vi "NavbalLabVIEW(15-5-21).vi"() -> ()   [LabVIEW 2010] (continued)
              n791 = Increment(x=w3724) -> (x+1=w3725:i32)
              n792 = local read "#Corner Accels"() -> (w3709:i32)
              n793 = Add(x=w3718, y=w3719) -> (x+y=w3720:i32)
              n794 = Add(x=12, y=w3720) -> (x+y=w3722:i32)
              n795 = Decrement(x=w3722) -> (x-1=w3717:i32)
              n796 = Bundle(w3717, w3725) -> (w3730:cluster{i32, i32})  [unwired: 1 in]
              n797 = call-poly <vilib>:"Excel Get Data.vi"("report in"=w3737, "data type"=string[][] [], "start (-1, -1)"=w3731, "end (-1, -1)"=w3730, "error in (no error)"=w3738) -> ("data"=w3729:string[][], "error out"=w3723:errorcluster)  [unwired: 9 out]
              n798 = call <vilib>:"General Error Handler.vi"("error in (no error)"=w3723) -> ()  [unwired: 2 in, 13 out]
              n799 = Fract/Exp String To Number(string=w3729) -> (number=w3710:dbl[][])  [unwired: 3 in, 1 out]
              n800 = case shown="\"Port Side\", Default" w3711 {
                tunnel: w3710 -> [w3752 w3766]
                tunnel: [w3744 w3757] -> w3712
                tunnel: w3709 -> [w3741 w3756]
                frame "Port Side", Default {
                  n801 = Initialize Array(0.0 ("element"), w3741, 2 ("dimension size")) -> (w3749:dbl[][])
                  n802 = Insert Into Array(array=w3752, index (row)=0, new element=w3749) -> (w3748:dbl[][])  [unwired: 1 in]
                  n803 = Multiply(x=2, y=w3741) -> (x*y=w3740:i32)
                  n804 = local read "#Stbd Accels"() -> (w3739:i32)
                  n805 = Initialize Array(0.0 ("element"), w3739, 2 ("dimension size")) -> (w3745:dbl[][])
                  n806 = Insert Into Array(array=w3748, index (row)=w3740, new element=w3745) -> (w3744:dbl[][])  [unwired: 1 in]
                }
                frame "Stbd Side" {
                  n807 = local read "#Stbd Accels"() -> (w3753:i32)
                  n808 = Initialize Array(0.0 ("element"), w3756, 2 ("dimension size")) -> (w3763:dbl[][])
                  n809 = Insert Into Array(array=w3766, index (row)=w3756, new element=w3763) -> (w3762:dbl[][])  [unwired: 1 in]
                  n810 = Multiply(x=2, y=w3756) -> (x*y=w3754:i32)
                  n811 = Add(x=w3754, y=w3753) -> (x+y=w3761:i32)
                  n812 = Initialize Array(0.0 ("element"), w3753, 2 ("dimension size")) -> (w3758:dbl[][])
                  n813 = Insert Into Array(array=w3762, index (row)=w3761, new element=w3758) -> (w3757:dbl[][])  [unwired: 1 in]
                }
              }
              "Ref Pt Plot" <- w3712
            }
          }
          n814 = case shown="True" "Refresh Plot Listbox" {
            tunnel: w3337 -> [_ w3779]
            frame False {
            }
            frame True {
              n815 = local read "Port/Starboard"() -> (w3782:enum32{"Port Side", "Stbd Side"})
              n816 = case shown="\"Port Side\", Default" w3782 {
                tunnel: ["Data-Port" "Data-Stbd"] -> w3781
                frame "Port Side", Default {
                }
                frame "Stbd Side" {
                }
              }
              n817 = call <vilib>:"New Report.vi"("report type"=T11."Excel", "template (empty)"=w3779) -> ("report out"=w3785:refnum<class "NI_report.lvclass">, "error out"=w3784:errorcluster)  [unwired: 12 in]
              n818 = call <vilib>:"Excel Get Worksheet.vi"("report in"=w3785, "error in (no error)"=w3784, "name (\"\")"=w3781) -> ("report out"=w3798:refnum<class "NI_report.lvclass">, "error out"=w3797:errorcluster)  [unwired: 1 in, 10 out]
              n819 = Increment(x="# Runs") -> (x+1=w3786:dbl)
              n820 = Multiply(x=w3786, y=2) -> (x*y=w3788:dbl)
              n821 = Bundle("row"=2, w3788) -> (w3787:cluster{"row":i32, dbl})  [unwired: 1 in]
              n822 = call-poly <vilib>:"Excel Get Data.vi"("report in"=w3798, "data type"=string[][] [], "start (-1, -1)"=cluster{"row":i32, "column":i32} {"row"=0, "column"=1}, "end (-1, -1)"=w3787, "error in (no error)"=w3797) -> ("data"=w3792:string[][])  [unwired: 10 out]
              n823 = Transpose 2D Array(2D array=w3792) -> (transposed array=w3795:string[][])
              n824 = local read "Predicted Phase"() -> (w3775:dbl[])
              n825 = Index Array(array=w3795, index (col)=0 ("disabled index (col)")) -> (element=w3794:string[])  [unwired: 1 in]
              n826 = Decimate 1D Array(w3794) -> (w3791:string[])  [unwired: 1 out]
              n827 = Array Size(array=w3791) -> (size(s)=w3793:i32)
              n828 = Reshape Array(w3791, w3793, 1 ("dimension size")) -> (w3783:string[][])
              n829 = local read "Predicted Mag"() -> (w3776:dbl[])
              n830 = local read "Select Side to Analyze"() -> (w3771:enum32{"Starboard", "Port"})
              n831 = property on="Marker Listbox" class="MCListbox (strict)"("ItemNames"=w3783) -> ()  [unwired: 2 in, 2 out]
              n832 = local read "#Corner Accels"() -> (w3773:i32)
              n833 = Build Array(w3776, w3775) -> (w3777:dbl[][])
              n834 = Transpose 2D Array(2D array=w3777) -> (transposed array=w3774:dbl[][])
              n835 = case shown="\"Port\"" w3771 {
                tunnel: w3774 -> [w3815 w3829]
                tunnel: [w3806 w3821] -> w3772
                tunnel: w3773 -> [w3805 w3818]
                frame "Starboard", Default {
                  n836 = local read "#Stbd Accels"() -> (w3802:i32)
                  n837 = Initialize Array(0.0 ("element"), w3805, 2 ("dimension size")) -> (w3812:dbl[][])
                  n838 = Insert Into Array(array=w3815, index (row)=w3805, new element=w3812) -> (w3811:dbl[][])  [unwired: 1 in]
                  n839 = Multiply(x=2, y=w3805) -> (x*y=w3803:i32)
                  n840 = Add(x=w3803, y=w3802) -> (x+y=w3810:i32)
                  n841 = Initialize Array(0.0 ("element"), w3802, 2 ("dimension size")) -> (w3807:dbl[][])
                  n842 = Insert Into Array(array=w3811, index (row)=w3810, new element=w3807) -> (w3806:dbl[][])  [unwired: 1 in]
                }
                frame "Port" {
                  n843 = Initialize Array(0.0 ("element"), w3818, 2 ("dimension size")) -> (w3826:dbl[][])
                  n844 = Insert Into Array(array=w3829, index (row)=0, new element=w3826) -> (w3825:dbl[][])  [unwired: 1 in]
                  n845 = Multiply(x=2, y=w3818) -> (x*y=w3817:i32)
                  n846 = local read "#Stbd Accels"() -> (w3816:i32)
                  n847 = Initialize Array(0.0 ("element"), w3816, 2 ("dimension size")) -> (w3822:dbl[][])
                  n848 = Insert Into Array(array=w3825, index (row)=w3817, new element=w3822) -> (w3821:dbl[][])  [unwired: 1 in]
                }
              }
              "Pred plot" <- w3772
            }
          }
          n849 = Divide(x=159.0, y=w3556) -> (x/y=w3700:dbl)
          n850 = Divide(x=159.0, y=w3557) -> (x/y=w3685:dbl)
          n851 = Logarithm Base 10(1:w3700) -> (0:w3699:dbl)
          n852 = Divide(x=159.0, y=w3643) -> (x/y=w3658:dbl)
          n853 = Logarithm Base 10(1:w3685) -> (0:w3684:dbl)
          n854 = Divide(x=159.0, y=w3483) -> (x/y=w3509:dbl)
          n855 = Multiply(x=20.0, y=w3699) -> (x*y=w3698:dbl)
          n856 = Logarithm Base 10(1:w3658) -> (0:w3657:dbl)
          n857 = Multiply(x=20.0, y=w3684) -> (x*y=w3683:dbl)
          n858 = Logarithm Base 10(1:w3509) -> (0:w3508:dbl)
          n859 = Subtract(x=w3696, y=w3698) -> (x-y=w3692:dbl[][])
          "Magnitude AdB Stbd" <- w3692
          n860 = Multiply(x=20.0, y=w3657) -> (x*y=w3656:dbl)
          n861 = Subtract(x=w3681, y=w3683) -> (x-y=w3674:dbl[][])
          "Magnitude AdB Port" <- w3674
          n862 = Multiply(x=20.0, y=w3508) -> (x*y=w3507:dbl)
          n863 = Subtract(x=w3644, y=w3656) -> (x-y=w3642:dbl[][])
          "Magnitude AdB Corner" <- w3642
          n864 = Subtract(x=w3495, y=w3507) -> (x-y=w3494:dbl[][])
          "Magnitude AdB Corners-Port" <- w3494
          n865 = local read "Averaging"() -> (w3365:bool)
          n866 = for "Mils(8x)" {
            N: w3521 -> [_]
            tunnel: w3696 -> [w5009]
            tunnel: w3556 -> [w5005]
            tunnel: [w5004] -> w3639 mode=indexing
            tunnel: [w5003] -> w3697 mode=indexing
            i -> [w5006]
            n867 = Index Array(array=w5009, index (row)=w5006) -> (element=w5007:dbl[])  [unwired: 1 in]
            n868 = for {
              N: 8 -> [_]
              tunnel: w5007 -> [w5018]
              tunnel: w5005 -> [w5026]
              tunnel: [w5012] -> w5004 mode=indexing
              tunnel: [w5010] -> w5003 mode=indexing
              i -> [w5025]
              n869 = Add(x=w5025, y=1) -> (x+y=w5027:i32)
              n870 = Index Array(array=w5018, index=w5025) -> (element=w5019:dbl)
              n871 = Multiply(x=w5026, y=w5027) -> (x*y=w5010:dbl)
              n872 = Divide(x=159, y=w5010) -> (x/y=w5023:dbl)
              n873 = Logarithm Base 10(1:w5023) -> (0:w5022:dbl)
              n874 = Multiply(x=20.0, y=w5022) -> (x*y=w5020:dbl)
              n875 = Subtract(x=w5019, y=w5020) -> (x-y=w5013:dbl)
              n876 = Divide(x=w5013, y=20.0) -> (x/y=w5015:dbl)
              n877 = Power Of 10(x=w5015) -> (10^x=w5017:dbl)
              n878 = Multiply(x=w5017, y=0.0887) -> (x*y=w5011:dbl)
              n879 = Divide(x=w5011, y=w5010) -> (x/y=w5012:dbl)
            }
          }
          "Mils/sec Stbd" <- w3639
          "Freq Stbd" <- w3697
          n880 = for "Mils(8x)" {
            N: w3519 -> [_]
            tunnel: w3681 -> [w4901]
            tunnel: w3557 -> [w4897]
            tunnel: [w4896] -> w3619 mode=indexing
            tunnel: [w4895] -> w3682 mode=indexing
            i -> [w4898]
            n881 = Index Array(array=w4901, index (row)=w4898) -> (element=w4899:dbl[])  [unwired: 1 in]
            n882 = for {
              N: 8 -> [_]
              tunnel: w4899 -> [w4910]
              tunnel: w4897 -> [w4918]
              tunnel: [w4904] -> w4896 mode=indexing
              tunnel: [w4902] -> w4895 mode=indexing
              i -> [w4917]
              n883 = Add(x=w4917, y=1) -> (x+y=w4919:i32)
              n884 = Index Array(array=w4910, index=w4917) -> (element=w4911:dbl)
              n885 = Multiply(x=w4918, y=w4919) -> (x*y=w4902:dbl)
              n886 = Divide(x=159, y=w4902) -> (x/y=w4915:dbl)
              n887 = Logarithm Base 10(1:w4915) -> (0:w4914:dbl)
              n888 = Multiply(x=20.0, y=w4914) -> (x*y=w4912:dbl)
              n889 = Subtract(x=w4911, y=w4912) -> (x-y=w4905:dbl)
              n890 = Divide(x=w4905, y=20.0) -> (x/y=w4907:dbl)
              n891 = Power Of 10(x=w4907) -> (10^x=w4909:dbl)
              n892 = Multiply(x=w4909, y=0.0887) -> (x*y=w4903:dbl)
              n893 = Divide(x=w4903, y=w4902) -> (x/y=w4904:dbl)
            }
          }
          "Mils/sec Port" <- w3619
          "Freq Port" <- w3682
          n894 = Index Array(array=w3692, index (col)=0 ("disabled index (col)")) -> (element=w3693:dbl[])  [unwired: 1 in]
          n895 = local read "Averaging"() -> (w3358:bool)
          n896 = for "Mils(8x)" {
            N: w3571 -> [_]
            tunnel: w3644 -> [w4713]
            tunnel: w3643 -> [w4709]
            tunnel: [w4708] -> w3617 mode=indexing
            tunnel: [w4707] -> w3655 mode=indexing
            i -> [w4710]
            n897 = Index Array(array=w4713, index (row)=w4710) -> (element=w4711:dbl[])  [unwired: 1 in]
            n898 = for {
              N: 8 -> [_]
              tunnel: w4711 -> [w4722]
              tunnel: w4709 -> [w4730]
              tunnel: [w4716] -> w4708 mode=indexing
              tunnel: [w4714] -> w4707 mode=indexing
              i -> [w4729]
              n899 = Add(x=w4729, y=1) -> (x+y=w4731:i32)
              n900 = Index Array(array=w4722, index=w4729) -> (element=w4723:dbl)
              n901 = Multiply(x=w4730, y=w4731) -> (x*y=w4714:dbl)
              n902 = Divide(x=159, y=w4714) -> (x/y=w4727:dbl)
              n903 = Logarithm Base 10(1:w4727) -> (0:w4726:dbl)
              n904 = Multiply(x=20.0, y=w4726) -> (x*y=w4724:dbl)
              n905 = Subtract(x=w4723, y=w4724) -> (x-y=w4717:dbl)
              n906 = Divide(x=w4717, y=20.0) -> (x/y=w4719:dbl)
              n907 = Power Of 10(x=w4719) -> (10^x=w4721:dbl)
              n908 = Multiply(x=w4721, y=0.0887) -> (x*y=w4715:dbl)
              n909 = Divide(x=w4715, y=w4714) -> (x/y=w4716:dbl)
            }
          }
          "Mils/sec Corner" <- w3617
          "Freq Corner" <- w3655
          n910 = Index Array(array=w3674, index (col)=0 ("disabled index (col)")) -> (element=w3678:dbl[])  [unwired: 1 in]
          n911 = for "Mils(8x)" {
            N: w3481 -> [_]
            tunnel: w3495 -> [w4264]
            tunnel: w3483 -> [w4260]
            tunnel: [w4259] -> w3485 mode=indexing
            tunnel: [w4258] -> w3506 mode=indexing
            i -> [w4261]
            n912 = Index Array(array=w4264, index (row)=w4261) -> (element=w4262:dbl[])  [unwired: 1 in]
            n913 = for {
              N: 8 -> [_]
              tunnel: w4262 -> [w4273]
              tunnel: w4260 -> [w4281]
              tunnel: [w4267] -> w4259 mode=indexing
              tunnel: [w4265] -> w4258 mode=indexing
              i -> [w4280]
              n914 = Add(x=w4280, y=1) -> (x+y=w4282:i32)
              n915 = Index Array(array=w4273, index=w4280) -> (element=w4274:dbl)
              n916 = Multiply(x=w4281, y=w4282) -> (x*y=w4265:dbl)
              n917 = Divide(x=159, y=w4265) -> (x/y=w4278:dbl)
              n918 = Logarithm Base 10(1:w4278) -> (0:w4277:dbl)
              n919 = Multiply(x=20.0, y=w4277) -> (x*y=w4275:dbl)
              n920 = Subtract(x=w4274, y=w4275) -> (x-y=w4268:dbl)
              n921 = Divide(x=w4268, y=20.0) -> (x/y=w4270:dbl)
              n922 = Power Of 10(x=w4270) -> (10^x=w4272:dbl)
              n923 = Multiply(x=w4272, y=0.0887) -> (x*y=w4266:dbl)
              n924 = Divide(x=w4266, y=w4265) -> (x/y=w4267:dbl)
            }
          }
          "Mils/sec Corners-Port" <- w3485
          "Freq Corner Port" <- w3506
          n925 = local read "Averaging"() -> (w3356:bool)
          n926 = local read "Averaging"() -> (w3357:bool)
          n927 = Index Array(array=w3642, index (col)=0 ("disabled index (col)")) -> (element=w3652:dbl[])  [unwired: 1 in]
          n928 = Array Size(array=w3693) -> (size(s)=w3695:i32)
          n929 = Index Array(array=w3494, index (col)=0 ("disabled index (col)")) -> (element=w3503:dbl[])  [unwired: 1 in]
          n930 = Index Array(array=w3639, index (col)=0 ("index (row)")) -> (element=w3363:dbl[])  [unwired: 1 in]
          n931 = Index Array(array=w3558, index (col)=0 ("index")) -> (element=w3364:dbl[])  [unwired: 1 in]
          n932 = Index Array(array=w3692, index (col)=0 ("index (row)")) -> (element=w3361:dbl[])  [unwired: 1 in]
          n933 = Array Size(array=w3678) -> (size(s)=w3680:i32)
          n934 = Index Array(array=w3619, index (col)=0 ("index (row)")) -> (element=w3675:dbl[])  [unwired: 1 in]
          n935 = case shown="True" w3365 {
            tunnel: [w3879 w3880] -> w3362
            tunnel: w3364 -> [w3879 w3881]
            frame False {
            }
            frame True {
              n936 = call "Time Averaging3"("input signals"=w3881) -> ("time avg. signal"=w3880:dbl[])  [unwired: 15 in, 3 out]
            }
          }
          n937 = Index Array(array=w3415, index (col)=0 ("index")) -> (element=w3414:dbl[])  [unwired: 1 in]
          n938 = Index Array(array=w3674, index (col)=0 ("index (row)")) -> (element=w3673:dbl[])  [unwired: 1 in]
          n939 = Array Size(array=w3652) -> (size(s)=w3654:i32)
          n940 = for "Mils(1x)" {
            N: w3695 -> [_]
            tunnel: w3556 -> [w4998]
            tunnel: [w4993] -> w3360 mode=indexing
            tunnel: w3693 -> [w4992]
            i -> [w5002]
            n941 = Square(x=w4998) -> (x^2=w4996:dbl)
            n942 = Index Array(array=w4992, index #1=w5002) -> (element #1=w5001:dbl)  [unwired: 1 in, 1 out]
            n943 = Divide(x=0.028175, y=w4996) -> (x/y=w4994:dbl)
            n944 = Divide(x=w5001, y=20.0) -> (x/y=w4999:dbl)
            n945 = Power Of 10(x=w4999) -> (10^x=w4995:dbl)
            n946 = Multiply(x=w4995, y=w4994) -> (x*y=w4993:dbl)
          }
          "Mils(1x) Stbd" <- w3360
          n947 = case shown="True" w3358 {
            tunnel: w3414 -> [w3876 w3878]
            tunnel: [w3876 w3877] -> w3408
            frame False {
            }
            frame True {
              n948 = call "Time Averaging2"("input signals"=w3878) -> ("time avg. signal"=w3877:dbl[])  [unwired: 15 in, 3 out]
            }
          }
          n949 = Index Array(array=w3617, index (col)=0 ("index (row)")) -> (element=w3649:dbl[])  [unwired: 1 in]
          n950 = Index Array(array=w3618, index (col)=0 ("index")) -> (element=w3413:dbl[])  [unwired: 1 in]
          n951 = Index Array(array=w3642, index (col)=0 ("index (row)")) -> (element=w3648:dbl[])  [unwired: 1 in]
          n952 = Array Size(array=w3503) -> (size(s)=w3505:i32)
          n953 = for "Mils(1x)" {
            N: w3680 -> [_]
            tunnel: w3557 -> [w4890]
            tunnel: [w4885] -> w3677 mode=indexing
            tunnel: w3678 -> [w4884]
            i -> [w4894]
            n954 = Square(x=w4890) -> (x^2=w4888:dbl)
            n955 = Index Array(array=w4884, index #1=w4894) -> (element #1=w4893:dbl)  [unwired: 1 in, 1 out]
            n956 = Divide(x=0.028175, y=w4888) -> (x/y=w4886:dbl)
            n957 = Divide(x=w4893, y=20.0) -> (x/y=w4891:dbl)
            n958 = Power Of 10(x=w4891) -> (10^x=w4887:dbl)
            n959 = Multiply(x=w4887, y=w4886) -> (x*y=w4885:dbl)
          }
          "Mils(1x) Port" <- w3677
          n960 = Index Array(array=w3485, index (col)=0 ("index (row)")) -> (element=w3500:dbl[])  [unwired: 1 in]
          n961 = Index Array(array=w3486, index (col)=0 ("index")) -> (element=w3411:dbl[])  [unwired: 1 in]
          n962 = case shown="True" w3356 {
            tunnel: w3411 -> [w3870 w3872]
            tunnel: [w3870 w3871] -> w3410
            frame False {
            }
            frame True {
              n963 = call "Time Averaging5"("input signals"=w3872) -> ("time avg. signal"=w3871:dbl[])  [unwired: 15 in, 3 out]
            }
          }
          n964 = Index Array(array=w3494, index (col)=0 ("index (row)")) -> (element=w3499:dbl[])  [unwired: 1 in]
          n965 = case shown="True" w3357 {
            tunnel: w3413 -> [w3873 w3875]
            tunnel: [w3873 w3874] -> w3412
            frame False {
            }
            frame True {
              n966 = call "Time Averaging4"("input signals"=w3875) -> ("time avg. signal"=w3874:dbl[])  [unwired: 15 in, 3 out]
            }
          }
          n967 = for "Mils(1x)" {
            N: w3654 -> [_]
            tunnel: w3643 -> [w4702]
            tunnel: [w4697] -> w3651 mode=indexing
            tunnel: w3652 -> [w4696]
            i -> [w4706]
            n968 = Square(x=w4702) -> (x^2=w4700:dbl)
            n969 = Index Array(array=w4696, index #1=w4706) -> (element #1=w4705:dbl)  [unwired: 1 in, 1 out]
            n970 = Divide(x=0.028175, y=w4700) -> (x/y=w4698:dbl)
            n971 = Divide(x=w4705, y=20.0) -> (x/y=w4703:dbl)
            n972 = Power Of 10(x=w4703) -> (10^x=w4699:dbl)
            n973 = Multiply(x=w4699, y=w4698) -> (x*y=w4697:dbl)
          }
          "Mils(1x) Corners" <- w3651
          n974 = for "Mils(1x)" {
            N: w3505 -> [_]
            tunnel: w3483 -> [w4253]
            tunnel: [w4248] -> w3502 mode=indexing
            tunnel: w3503 -> [w4247]
            i -> [w4257]
            n975 = Square(x=w4253) -> (x^2=w4251:dbl)
            n976 = Index Array(array=w4247, index #1=w4257) -> (element #1=w4256:dbl)  [unwired: 1 in, 1 out]
            n977 = Divide(x=0.028175, y=w4251) -> (x/y=w4249:dbl)
            n978 = Divide(x=w4256, y=20.0) -> (x/y=w4254:dbl)
            n979 = Power Of 10(x=w4254) -> (10^x=w4250:dbl)
            n980 = Multiply(x=w4250, y=w4249) -> (x*y=w4248:dbl)
          }
          "Mils(1x) Corners-Port" <- w3502
          n981 = Build Array(w3363, w3362, w3361, w3360) -> (w3359:dbl[][])
          n982 = Build Array(w3675, w3408, w3673, w3677) -> (w3676:dbl[][])
          n983 = Build Array(w3649, w3412, w3648, w3651) -> (w3650:dbl[][])
          n984 = Build Array(w3500, w3410, w3499, w3502) -> (w3501:dbl[][])
          n985 = Transpose Matrix(1:w3359) -> (0:→"Starboard Arrays":dbl[][])
          n986 = Transpose Matrix(1:w3676) -> (0:→"Port Arrays":dbl[][])
          n987 = Transpose Matrix(1:w3650) -> (0:→"Corner Arrays Stbd":dbl[][])
          n988 = Transpose Matrix(1:w3501) -> (0:→"Corner Arrays Port":dbl[][])
          n989 = call <vilib>:"Value Has Changed PtByPt.vi"("input data point"=w3329) -> ("has changed"=w3341:bool)  [unwired: 1 in, 1 out]
          n990 = Or(x="Clear Save array", y=w3341) -> (x .or. y?=w3342:bool)
          n991 = Array Subset(array=w3639, index (col)=0 ("index"), length (col)=1 ("length")) -> (w3636:dbl[][])  [unwired: 2 in]
          n992 = Array Subset(array=w3558, index (col)=0 ("index"), length (col)=1 ("length")) -> (w3634:dbl[][])  [unwired: 2 in]
          n993 = case shown="True" w3342 {
            tunnel: w3329 -> [_ w3837]
            frame False {
            }
            frame True {
              n994 = local read "# of Runs to include"() -> (w3833:i32)
              n995 = local read "Boat File"() -> (w3840:path)
              n996 = case shown="\"Port Side\", Default" w3837 {
                tunnel: ["Data-Port" "Data-Stbd"] -> w3842
                frame "Port Side", Default {
                }
                frame "Stbd Side" {
                }
              }
              n997 = Multiply(x=w3833, y=2) -> (x*y=w3832:i32)
              n998 = call <vilib>:"New Report.vi"("report type"=T11."Excel", "template (empty)"=w3840) -> ("report out"=w3844:refnum<class "NI_report.lvclass">, "error out"=w3843:errorcluster)  [unwired: 12 in]
              n999 = call <vilib>:"Excel Get Worksheet.vi"("report in"=w3844, "error in (no error)"=w3843, "name (\"\")"=w3842) -> ("report out"=w3846:refnum<class "NI_report.lvclass">, "error out"=w3845:errorcluster)  [unwired: 1 in, 10 out]
              n1000 = Bundle("row"=0, w3832) -> (w3835:cluster{"row":i32, i32})  [unwired: 1 in]
              n1001 = call-poly <vilib>:"Excel Get Data.vi"("report in"=w3846, "data type"=string[][] [], "start (-1, -1)"=cluster{"row":i32, "column":i32} {"row"=0, "column"=1}, "end (-1, -1)"=w3835, "error in (no error)"=w3845) -> ("data"=w3848:string[][])  [unwired: 10 out]
              n1002 = Index Array(array=w3848, index (row)=0) -> (element=w3849:string[])  [unwired: 1 in]
              n1003 = Decimate 1D Array(w3849) -> (w3850:string[])  [unwired: 1 out]
              n1004 = local write "Weight+Location"(dbl[][] [[0.0, 0.0, 0.0, 0.0], [0.0, 0.0, 0.0, 0.0], [0.0, 0.0, 0.0, 0.0], [0.0, 0.0, 0.0, 0.0]] ("Weight+Location")) -> ()
              n1005 = property on="Run Reference:" class="Ring (strict)"("Strings []"=w3850) -> ()  [unwired: 2 in, 2 out]
            }
          }
          n1006 = Array Subset(array=w3617, index (col)=0 ("index"), length (col)=1 ("length")) -> (w3622:dbl[][])  [unwired: 2 in]
          n1007 = Array Subset(array=w3618, index (col)=0 ("index"), length (col)=1 ("length")) -> (w3620:dbl[][])  [unwired: 2 in]
          n1008 = Array Subset(array=w3485, index (col)=0 ("index"), length (col)=1 ("length")) -> (w3489:dbl[][])  [unwired: 2 in]
          n1009 = Insert Into Array(array=w3636, index (col)=1 ("disabled index (col)"), new element=w3634) -> (w3440:dbl[][])  [unwired: 1 in]
          "Mils/Sec-Phase(STBD)" <- w3440
          n1010 = Array Subset(array=w3486, index (col)=0 ("index"), length (col)=1 ("length")) -> (w3487:dbl[][])  [unwired: 2 in]
          n1011 = Insert Into Array(array=w3622, index (col)=1 ("disabled index (col)"), new element=w3620) -> (w3438:dbl[][])  [unwired: 1 in]
          "Mils/Sec-Phase(CORNERS-Stbd)" <- w3438
          n1012 = Insert Into Array(array=w3489, index (col)=1 ("disabled index (col)"), new element=w3487) -> (w3437:dbl[][])  [unwired: 1 in]
          "Mils/Sec-Phase(CORNERS-Port)" <- w3437
          n1013 = Array Subset(array=w3619, index (col)=0 ("index"), length (col)=1 ("length")) -> (w3629:dbl[][])  [unwired: 2 in]
          n1014 = Array Subset(array=w3415, index (col)=0 ("index"), length (col)=1 ("length")) -> (w3627:dbl[][])  [unwired: 2 in]
          n1015 = case shown="True" "Clear Strtpt" {
            frame False {
            }
            frame True {
              n1016 = local write "Ref Pt Plot"(dbl[][] [] ("Weight+Location")) -> ()
              n1017 = local write "Indicate Ref"("" ("Indicate Ref")) -> ()
            }
          }
          n1018 = Insert Into Array(array=w3629, index (col)=1 ("disabled index (col)"), new element=w3627) -> (w3439:dbl[][])  [unwired: 1 in]
          "Mils/Sec-Phase(PORT)" <- w3439
          n1019 = case "Saving run - Data Acquisition Tab" shown="True" "Save Run" {
            frame False {
            }
            frame True {
              w4625 = -4142 items=["xlRangeAutoFormat3DEffects1"=13, "xlRangeAutoFormat3DEffects2"=14, "xlRangeAutoFormatAccounting1"=4, "xlRangeAutoFormatAccounting2"=5, "xlRangeAutoFormatAccounting3"=6, "xlRangeAutoFormatAccounting4"=17, "xlRangeAutoFormatClassic1"=1, "xlRangeAutoFormatClassic2"=2, "xlRangeAutoFormatClassic3"=3, "xlRangeAutoFormatColor1"=7, "xlRangeAutoFormatColor2"=8, "xlRangeAutoFormatColor3"=9, "xlRangeAutoFormatList1"=10, "xlRangeAutoFormatList2"=11, "xlRangeAutoFormatList3"=12, "xlRangeAutoFormatLocalFormat1"=15, "xlRangeAutoFormatLocalFormat2"=16, "xlRangeAutoFormatLocalFormat3"=19, "xlRangeAutoFormatLocalFormat4"=20, "xlRangeAutoFormatReport1"=21, "xlRangeAutoFormatReport2"=22, "xlRangeAutoFormatReport3"=23, "xlRangeAutoFormatReport4"=24, "xlRangeAutoFormatReport5"=25, "xlRangeAutoFormatReport6"=26, "xlRangeAutoFormatReport7"=27, "xlRangeAutoFormatReport8"=28, "xlRangeAutoFormatReport9"=29, "xlRangeAutoFormatReport10"=30, "xlRangeAutoFormatClassicPivotTable"=31, "xlRangeAutoFormatTable1"=32, "xlRangeAutoFormatTable2"=33, "xlRangeAutoFormatTable3"=34, "xlRangeAutoFormatTable4"=35, "xlRangeAutoFormatTable5"=36, "xlRangeAutoFormatTable6"=37, "xlRangeAutoFormatTable7"=38, "xlRangeAutoFormatTable8"=39, "xlRangeAutoFormatTable9"=40, "xlRangeAutoFormatTable10"=41, "xlRangeAutoFormatPTNone"=42, "xlRangeAutoFormatNone"=-4142, "xlRangeAutoFormatSimple"=-4154] ("auto format (none)")
              w4614 = u16 3 items=["shift cells right", "shift cells down", "entire row", "entire column"] ("mode (entire row)")
              w4615 = cluster{"row":i32, "column":i32} {"row"=0, "column"=1} ("start (-1, -1)")
              w4543 = T18 {"font name"="Calibri", "font size"=12.0, "bold"=0, "italic"=0, "underline"=0, "strike through"=0, "font color"=0} ("font")
              # "4 planes"
              n1020 = local read "Divisions in\nEach Plane"() -> (w4584:T3)
              n1021 = Number To Fractional String(number="Weight+Location", precision (6)=i16 2) -> (F-format string=w4578:string[][])  [unwired: 2 in]
              n1022 = local read "time string"() -> (w4563:string)
              n1023 = Transpose 2D Array(2D array=w4578) -> (transposed array=w4573:string[][])
              n1024 = Index Array(array=w4584, index (col)=0 ("disabled index (col)")) -> (element=w4582:dbl[])  [unwired: 1 in]
              n1025 = for {
                N: 4 -> [_]
                tunnel: "Weight+Location" -> [w4689]
                tunnel: w4582 -> [w4667] mode=indexing
                tunnel: [w4655] -> w4581 mode=indexing
                tunnel: [w4653] -> w4580 mode=indexing
                i -> [w4688]
                n1026 = Index Array "Pick Plane"(array=w4689, index (row)=w4688) -> (element=w4683:dbl[])  [unwired: 1 in]
                n1027 = Index Array "Pick Mag"(array=w4683, index=0) -> (element=w4682:dbl)
                n1028 = Index Array "Pick Loc"(array=w4683, index=1) -> (element=w4681:dbl)
                n1029 = Index Array "Pick Mag"(array=w4683, index=2) -> (element=w4665:dbl)
                n1030 = Index Array "Pick Loc"(array=w4683, index=3) -> (element=w4668:dbl)
                n1031 = Decrement(x=w4681) -> (x-1=w4680:dbl)
                n1032 = Decrement(x=w4668) -> (x-1=w4669:dbl)
                n1033 = Divide(x=360.0, y=w4667) -> (x/y=w4647:dbl)
                n1034 = Multiply(x=w4647, y=w4680) -> (x*y=w4678:dbl)
                n1035 = Multiply(x=w4647, y=w4669) -> (x*y=w4670:dbl)
                n1036 = Multiply(x=w4678, y=3.141592653589793) -> (x*y=w4676:dbl)
                n1037 = Multiply(x=w4670, y=3.141592653589793) -> (x*y=w4672:dbl)
                n1038 = Divide(x=w4676, y=180.0) -> (x/y=w4674:dbl)
                n1039 = Divide(x=w4672, y=180.0) -> (x/y=w4666:dbl)
                n1040 = Polar To Complex(1:w4674, 2:w4682) -> (0:w4664:cdb)
                n1041 = Polar To Complex(1:w4666, 2:w4665) -> (0:w4663:cdb)
                n1042 = Add(x=w4664, y=w4663) -> (x+y=w4662:cdb)
                n1043 = Complex To Polar(r * e^(i*theta)=w4662) -> (r=w4654:dbl, theta=w4649:dbl)
                n1044 = Greater Or Equal To 0?(x=w4649) -> (x >= 0?=w4650:bool)
                n1045 = Add(x=w4649, y=6.283185307179586) -> (x+y=w4651:dbl)
                n1046 = Select(t=w4649, s=w4650, f=w4651) -> (s? t:f=w4648:dbl)
                n1047 = Multiply(x=w4648, y=180.0) -> (x*y=w4660:dbl)
                n1048 = Divide(x=w4660, y=3.141592653589793) -> (x/y=w4658:dbl)
                n1049 = Divide(x=w4658, y=w4647) -> (x/y=w4657:dbl)
                n1050 = Increment(x=w4657) -> (x+1=w4656:dbl)
                n1051 = Number To Fractional String(number=w4654) -> (F-format string=w4653:string)  [unwired: 3 in]
                n1052 = Number To Fractional String(number=w4656) -> (F-format string=w4655:string)  [unwired: 3 in]
              }
              n1053 = local read "date string"() -> (w4565:string)
              n1054 = Index Array(array=w4573, index (row)=0) -> (element=w4572:string[])  [unwired: 1 in]
              n1055 = Index Array(array=w4573, index (row)=1) -> (element=w4571:string[])  [unwired: 1 in]
              n1056 = Index Array(array=w4573, index (row)=2) -> (element=w4570:string[])  [unwired: 1 in]
              n1057 = Index Array(array=w4573, index (row)=3) -> (element=w4569:string[])  [unwired: 1 in]
              n1058 = for {
                tunnel: w4572 -> [w4627] mode=indexing
                tunnel: w4571 -> [w4629] mode=indexing
                tunnel: w4570 -> [w4631] mode=indexing
                tunnel: w4569 -> [w4634] mode=indexing
                tunnel: [w4636] -> w4568 mode=indexing
                tunnel: [w4635] -> w4567 mode=indexing
                n1059 = Equal?(x=w4627, y="0.00") -> (x = y?=w4628:bool)
                n1060 = Equal?(x=w4631, y="0.00") -> (x = y?=w4633:bool)
                n1061 = case shown="False" w4628 {
                  tunnel: w4627 -> [w4640 _]
                  tunnel: w4629 -> [w4639 _]
                  tunnel: [w4638 "" ("y")] -> w4636
                  frame False {
                    n1062 = Concatenate Strings(w4640, " @" ("string"), w4639) -> (w4638:string)
                  }
                  frame True {
                  }
                }
                n1063 = case shown="True" w4633 {
                  tunnel: w4631 -> [w4645 _]
                  tunnel: w4634 -> [w4644 _]
                  tunnel: [w4643 "" ("y")] -> w4635
                  frame False {
                    n1064 = Concatenate Strings(w4645, " @" ("string"), w4644) -> (w4643:string)
                  }
                  frame True {
                  }
                }
              }
              n1065 = Build Array("Save Run As:", w4565, w4563) -> (w4562:string[])
              n1066 = Build Array(w4568, w4567) -> (w4558:string[][])
              n1067 = Insert Into Array(array=string[][] [], index (row)=0, new element=w4562) -> (w4559:string[][])  [unwired: 1 in]
              n1068 = local read "Boat File"() -> (w4545:path)
              n1069 = Insert Into Array(array=w4558, index (col)=0 ("disabled index (col)"), new element=w4559) -> (w4546:string[][])  [unwired: 1 in]
              n1070 = case shown="\"Port Side\", Default" "Port/Starboard" {
                tunnel: ["Data-Port" "Data-Stbd"] -> w4591
                tunnel: ["Data-PortLog" ("name (\"\")") "Data-StbdLog" ("name (\"\")")] -> w4544
                frame "Port Side", Default {
                }
                frame "Stbd Side" {
                }
              }
              n1071 = Multiply(x="# of Runs to include", y=2) -> (x*y=w4528:i32)
              n1072 = call <vilib>:"New Report.vi"("report type"=T11."Excel", "template (empty)"=w4545) -> ("report out"=w4541:refnum<class "NI_report.lvclass">, "error out"=w4540:errorcluster)  [unwired: 12 in]
              n1073 = Bundle("row"=0, w4528) -> (w4529:cluster{"row":i32, i32})  [unwired: 1 in]
              n1074 = call <vilib>:"Excel Get Worksheet.vi"("report in"=w4541, "error in (no error)"=w4540, "name (\"\")"=w4591) -> ("report out"=w4535:refnum<class "NI_report.lvclass">, "error out"=w4534:errorcluster)  [unwired: 1 in, 10 out]
              n1075 = Array Size(array=w4581) -> (size(s)=w4605:i32)
              n1076 = call <vilib>:"Excel Get Worksheet.vi"("report in"=w4541, "error in (no error)"=w4540, "name (\"\")"=w4544) -> ("report out"=w4555:refnum<class "NI_report.lvclass">, "error out"=w4554:errorcluster)  [unwired: 1 in, 10 out]
              n1077 = call-poly <vilib>:"Excel Get Data.vi"("report in"=w4535, "data type"=string[][] [], "start (-1, -1)"=cluster{"row":i32, "column":i32} {"row"=0, "column"=1}, "end (-1, -1)"=w4529, "error in (no error)"=w4534) -> ("data"=w4539:string[][])  [unwired: 10 out]
              n1078 = call <vilib>:"Excel Get Last Row.vi"("report in"=w4555, "error in (no error)"=w4554) -> ("report out"=w4549:refnum<class "NI_report.lvclass">, "MS Office parameters out"=w4553:T14, "error out"=w4548:errorcluster)  [unwired: 11 in]
              n1079 = Reshape Array(w4581, w4605, 1 ("dimension size")) -> (w4604:string[][])
              n1080 = Unbundle(w4553) -> ("position (Excel)"=w4552:cluster{"row":i32, "column":i32})  [unwired: 2 out]
              n1081 = call <vilib>:"Excel Insert Cells.vi"("report in"=w4535, "mode (entire row)"=w4614, "start (0, 0)"=w4615, "error in (no error)"=w4534) -> ("report out"=w4617:refnum<class "NI_report.lvclass">, "error out"=w4616:errorcluster)  [unwired: 10 in]
              n1082 = Index Array(array=w4539, index (row)=0) -> (element=w4536:string[])  [unwired: 1 in]
              n1083 = Unbundle(w4552) -> ("row"=w4550:i32)  [unwired: 1 out]
              n1084 = call <vilib>:"Excel Insert Cells.vi"("report in"=w4617, "mode (entire row)"=w4614, "start (0, 0)"=w4615, "error in (no error)"=w4616) -> ("report out"=w4587:refnum<class "NI_report.lvclass">, "error out"=w4586:errorcluster)  [unwired: 10 in]
              n1085 = Decimate 1D Array(w4536) -> (w4532:string[])  [unwired: 1 out]
              n1086 = Index Array(array=w4532, index="Run Reference:") -> (element=w4531:string)
              n1087 = Build Array (concatenate)("Save Run As:", w4565, w4563, w4531, "Mag (mils/s)", w4580) -> (w4566:string[])
              n1088 = Array Size(array=w4566) -> (size(s)=w4603:i32)
              n1089 = Reshape Array(w4566, w4603, 1 ("dimension size")) -> (w4593:string[][])
              n1090 = Replace Array Subset(array=w4593, new element="Phase (deg)", index (row)=4 ("disabled index (col)"), index (col)=0 ("index")) -> (w4597:string[][])
              n1091 = Delete From Array(array=w4597, length=8, index (row)=5 ("disabled index (col)")) -> (array with subset deleted=w4596:string[][])  [unwired: 1 in, 1 out]
              n1092 = Build Array (concatenate)(w4596, w4604) -> (w4594:string[][])
              n1093 = Bundle("row"=w4550, "index"=0) -> (w4547:cluster{"row":i32, "index":i32})  [unwired: 1 in]
              n1094 = Insert Into Array(array=w4593, index (col)=1 ("disabled index (col)"), new element=w4594) -> (w4592:string[][])  [unwired: 1 in]
              "Excel Output Array" <- w4592
              n1095 = call-poly <vilib>:"Excel Easy Table.vi"("report in"=w4549, "font"=w4543, "start (0, 0)"=w4547, "text data"=w4546, "error in (no error)"=w4548) -> ()  [unwired: 6 in, 5 out]
              n1096 = call-poly <vilib>:"Excel Easy Table.vi"("report in"=w4587, "font"=w4543, "auto format (none)"=w4625, "start (0, 0)"=w4615, "text data"=w4592, "error in (no error)"=w4586) -> ("report out"=w4624:refnum<class "NI_report.lvclass">, "error out"=w4623:errorcluster)  [unwired: 5 in, 3 out]
              n1097 = case shown="\"Port Side\", Default" "Port/Starboard" {
                tunnel: [w4690 w4691] -> w4613
                frame "Port Side", Default {
                  n1098 = local read "Port Output Data"() -> (w4690:string[][])
                }
                frame "Stbd Side" {
                  n1099 = local read "Stbd Output Data"() -> (w4691:string[][])
                }
              }
              n1100 = Array Size(array=w4613) -> (size(s)=w4612:i32[])
              n1101 = Index Array(array=w4612, index=0) -> (element=w4610:i32)
              n1102 = Array Subset(array=w4613, index (row)=0 ("index"), length (row)=w4610, index (col)=1 ("length"), length (col)=2 ("length")) -> (w4590:string[][])
              n1103 = Array Subset(array=w4590) -> (w4588:string[][])  [unwired: 4 in]
              n1104 = call-poly <vilib>:"Excel Easy Table.vi"("report in"=w4624, "font"=w4543, "start (0, 0)"=cluster{"row":i32, "column":i32} {"row"=12, "column"=1} ("start (-1, -1)"), "text data"=w4588, "error in (no error)"=w4623) -> ("report out"=w4622:refnum<class "NI_report.lvclass">, "error out"=w4621:errorcluster)  [unwired: 6 in, 3 out]
              n1105 = call-dynamic "Save Report to File.vi"("report in"=w4622, "report file path"=w4545, "error in (no error)"=w4621) -> ()  [unwired: 11 in, 2 out]
            }
          }
          n1106 = Build Array (concatenate)(w3440, w3434) -> (w3474:dbl[][][])
          n1107 = Build Array (concatenate)(w3439, w3433) -> (w3344:dbl[][][])
          n1108 = Build Array (concatenate)(w3438, w3432) -> (w3473:dbl[][][])
          n1109 = Build Array (concatenate)(w3437, w3431) -> (w3472:dbl[][][])
          n1110 = for "Magnitude (AdB)" {
            N: w3571 -> [_]
            tunnel: w3480 -> [w4036]
            tunnel: [w4032] -> w3404 mode=indexing
            i -> [w4035]
            n1111 = Index Array(array=w4036, index=w4035) -> (element=w4030:cluster{"x0":dbl, "dx":dbl, "magnitude":dbl[]})
            n1112 = Unbundle(w4030) -> ("dx"=w4031:dbl, "magnitude"=w4033:dbl[])  [unwired: 1 out]
            n1113 = Array Size(array=w4033) -> (size(s)=w4034:i32)
            n1114 = for {
              N: w4034 -> [_]
              tunnel: w4031 -> [w4047]
              tunnel: w4033 -> [w4045]
              tunnel: [w4038] -> w4032 mode=indexing
              i -> [w4046]
              n1115 = Index Array(array=w4045, index=w4046) -> (element=w4037:dbl)
              n1116 = Multiply(x=w4047, y=w4046) -> (x*y=w4039:dbl)
              n1117 = Divide(x=159, y=w4039) -> (x/y=w4042:dbl)
              n1118 = Logarithm Base 10(1:w4042) -> (0:w4043:dbl)
              n1119 = Multiply(x=20.0, y=w4043) -> (x*y=w4040:dbl)
              n1120 = Subtract(x=w4037, y=w4040) -> (x-y=w4038:dbl)
            }
          }
          n1121 = for "Magnitude (AdB)" {
            N: w3521 -> [_]
            tunnel: w3478 -> [w4074]
            tunnel: [w4072] -> w3403 mode=indexing
            i -> [w4068]
            n1122 = Increment(x=w4068) -> (x+1=w4067:i32)
            n1123 = Index Array(array=w4074, index=w4067) -> (element=w4070:cluster{"x0":dbl, "dx":dbl, "magnitude":dbl[]})
            n1124 = Unbundle(w4070) -> ("dx"=w4071:dbl, "magnitude"=w4073:dbl[])  [unwired: 1 out]
            n1125 = Array Size(array=w4073) -> (size(s)=w4069:i32)
            n1126 = for {
              N: w4069 -> [_]
              tunnel: w4071 -> [w4085]
              tunnel: w4073 -> [w4083]
              tunnel: [w4076] -> w4072 mode=indexing
              i -> [w4084]
              n1127 = Index Array(array=w4083, index=w4084) -> (element=w4075:dbl)
              n1128 = Multiply(x=w4085, y=w4084) -> (x*y=w4077:dbl)
              n1129 = Divide(x=159, y=w4077) -> (x/y=w4080:dbl)
              n1130 = Logarithm Base 10(1:w4080) -> (0:w4081:dbl)
              n1131 = Multiply(x=20.0, y=w4081) -> (x*y=w4078:dbl)
              n1132 = Subtract(x=w4075, y=w4078) -> (x-y=w4076:dbl)
            }
          }
          n1133 = for "Magnitude (AdB)" {
            N: w3519 -> [_]
            tunnel: w3523 -> [w4055]
            tunnel: [w4053] -> w3402 mode=indexing
            i -> [w4049]
            n1134 = Increment(x=w4049) -> (x+1=w4048:i32)
            n1135 = Index Array(array=w4055, index=w4048) -> (element=w4051:cluster{"x0":dbl, "dx":dbl, "magnitude":dbl[]})
            n1136 = Unbundle(w4051) -> ("dx"=w4052:dbl, "magnitude"=w4050:dbl[])  [unwired: 1 out]
            n1137 = Array Size(array=w4050) -> (size(s)=w4054:i32)
            n1138 = for {
              N: w4054 -> [_]
              tunnel: w4052 -> [w4066]
              tunnel: w4050 -> [w4064]
              tunnel: [w4057] -> w4053 mode=indexing
              i -> [w4065]
              n1139 = Index Array(array=w4064, index=w4065) -> (element=w4056:dbl)
              n1140 = Multiply(x=w4066, y=w4065) -> (x*y=w4058:dbl)
              n1141 = Divide(x=159, y=w4058) -> (x/y=w4061:dbl)
              n1142 = Logarithm Base 10(1:w4061) -> (0:w4062:dbl)
              n1143 = Multiply(x=20.0, y=w4062) -> (x*y=w4059:dbl)
              n1144 = Subtract(x=w4056, y=w4059) -> (x-y=w4057:dbl)
            }
          }
          n1145 = property on="Tab 2" class="TabCtl (strict)"() -> ("Value"=w3454:T1)  [unwired: 2 in, 2 out]
          n1146 = property on="Tab 2" class="TabCtl (strict)"() -> ("Visible"=w3451:bool)  [unwired: 2 in, 2 out]
          n1147 = local read "#Corner Accels"() -> (w3373:i32)
          n1148 = local read "Sensor Info"() -> (w3471:string[][])
          n1149 = local read "#Stbd Accels"() -> (w3372:i32)
          n1150 = Less Or Equal?(x=w3454, y=T20."Step 4: Background Checks") -> (x <= y?=w3452:bool)
          n1151 = local read "#Port Accels"() -> (w3370:i32)
          n1152 = And(x=w3452, y=w3451) -> (x .and. y?=w3450:bool)
          n1153 = Index Array(array=w3478, index=0) -> (element=w3465:cluster{"x0":dbl, "dx":dbl, "magnitude":dbl[]})
          n1154 = Index Array(array=w3523, index=0) -> (element=w3469:cluster{"x0":dbl, "dx":dbl, "magnitude":dbl[]})
          n1155 = Index Array(array=w3480, index=0) -> (element=w3461:cluster{"x0":dbl, "dx":dbl, "magnitude":dbl[]})
          n1156 = Unbundle(w3465) -> ("x0"=w3464:dbl, "dx"=w3463:dbl)  [unwired: 1 out]
          n1157 = Unbundle(w3469) -> ("x0"=w3468:dbl, "dx"=w3467:dbl)  [unwired: 1 out]
          n1158 = Add(x=w3373, y=w3372) -> (x+y=w3371:i32)
          n1159 = Unbundle(w3461) -> ("x0"=w3460:dbl, "dx"=w3459:dbl)  [unwired: 1 out]
          n1160 = case shown="True" "Save Vibration Survey" {
            tunnel: w3404 -> [_ w3923]
            tunnel: w3403 -> [_ w3922]
            tunnel: w3402 -> [_ w3921]
            frame False {
            }
            frame True {
              w3917 = -4142 items=["xlRangeAutoFormat3DEffects1"=13, "xlRangeAutoFormat3DEffects2"=14, "xlRangeAutoFormatAccounting1"=4, "xlRangeAutoFormatAccounting2"=5, "xlRangeAutoFormatAccounting3"=6, "xlRangeAutoFormatAccounting4"=17, "xlRangeAutoFormatClassic1"=1, "xlRangeAutoFormatClassic2"=2, "xlRangeAutoFormatClassic3"=3, "xlRangeAutoFormatColor1"=7, "xlRangeAutoFormatColor2"=8, "xlRangeAutoFormatColor3"=9, "xlRangeAutoFormatList1"=10, "xlRangeAutoFormatList2"=11, "xlRangeAutoFormatList3"=12, "xlRangeAutoFormatLocalFormat1"=15, "xlRangeAutoFormatLocalFormat2"=16, "xlRangeAutoFormatLocalFormat3"=19, "xlRangeAutoFormatLocalFormat4"=20, "xlRangeAutoFormatReport1"=21, "xlRangeAutoFormatReport2"=22, "xlRangeAutoFormatReport3"=23, "xlRangeAutoFormatReport4"=24, "xlRangeAutoFormatReport5"=25, "xlRangeAutoFormatReport6"=26, "xlRangeAutoFormatReport7"=27, "xlRangeAutoFormatReport8"=28, "xlRangeAutoFormatReport9"=29, "xlRangeAutoFormatReport10"=30, "xlRangeAutoFormatClassicPivotTable"=31, "xlRangeAutoFormatTable1"=32, "xlRangeAutoFormatTable2"=33, "xlRangeAutoFormatTable3"=34, "xlRangeAutoFormatTable4"=35, "xlRangeAutoFormatTable5"=36, "xlRangeAutoFormatTable6"=37, "xlRangeAutoFormatTable7"=38, "xlRangeAutoFormatTable8"=39, "xlRangeAutoFormatTable9"=40, "xlRangeAutoFormatTable10"=41, "xlRangeAutoFormatPTNone"=42, "xlRangeAutoFormatNone"=-4142, "xlRangeAutoFormatSimple"=-4154] ("auto format (none)")
              w3893 = 1921 ("length")
              # "Collect from 10Hz - 490Hz\nThis will encompass 8 \nrotationals"
              n1161 = local read "Boat File"() -> (w3919:path)
              n1162 = Build Array (concatenate)(w3923, w3922, w3921) -> (w3920:dbl[][])
              n1163 = call <vilib>:"New Report.vi"("report type"=T11."Excel", "template (empty)"=w3919) -> ("report out"=w3905:refnum<class "NI_report.lvclass">, "error out"=w3904:errorcluster)  [unwired: 12 in]
              n1164 = call <vilib>:"Excel Add Worksheet.vi"("report in"=w3905, "error in (no error)"=w3904) -> ("report out"=w3903:refnum<class "NI_report.lvclass">, "error out"=w3902:errorcluster)  [unwired: 12 in]
              n1165 = Transpose 2D Array(2D array=w3920) -> (transposed array=w3927:dbl[][])
              n1166 = call <vilib>:"Excel Workbook Properties.vi"("report in"=w3903, "error in (no error)"=w3902) -> ("report out"=w3912:refnum<class "NI_report.lvclass">, "worksheets count"=w3901:i32, "error out"=w3911:errorcluster)  [unwired: 10 in, 1 out]
              n1167 = Decrement(x=w3901) -> (x-1=w3900:i32)
              n1168 = Array Subset(array=w3927, index (row)=40 ("index"), length (row)=w3893) -> (w3924:dbl[][])  [unwired: 2 in]
              n1169 = for {
                N: w3893 -> [_]
                tunnel: [w3928] -> w3891 mode=indexing
                i -> [w3934]
                n1170 = Multiply(x=0.25, y=w3934) -> (x*y=w3932:dbl)
                n1171 = Add(x=10.0, y=w3932) -> (x+y=w3929:dbl)
                n1172 = Number To Fractional String(number=w3929, precision (6)=i16 3 ("width (-)")) -> (F-format string=w3928:string)  [unwired: 2 in]
              }
              n1173 = call <vilib>:"Excel Get Worksheet.vi"("report in"=w3912, "worksheet index (0)"=w3900, "error in (no error)"=w3911) -> ("report out"=w3910:refnum<class "NI_report.lvclass">, "error out"=w3909:errorcluster)  [unwired: 11 out]
              n1174 = call <vilib>:"Excel Rename Worksheet.vi"("report in"=w3910, "worksheet name (\"\")"="Vibration Survey Name", "error in (no error)"=w3909) -> ("report out"=w3908:refnum<class "NI_report.lvclass">, "error out"=w3907:errorcluster)  [unwired: 11 in]
              n1175 = Number To Fractional String(number=w3924, precision (6)=i16 3 ("width (-)")) -> (F-format string=w3884:string[][])  [unwired: 2 in]
              n1176 = Insert Into Array(array=w3884, index (col)=0 ("disabled index (col)"), new element=w3891) -> (w3883:string[][])  [unwired: 1 in]
              n1177 = local read "# Accel Channels"() -> (w3897:i32)
              n1178 = local read "Sensor Info"() -> (w3899:string[][])
              n1179 = Array Subset(array=w3899, index (row)=0 ("index"), length (row)=w3897, index (col)=0 ("index"), length (col)=1 ("length")) -> (w3890:string[][])
              n1180 = Index Array(array=w3890, index (col)=0 ("disabled index (col)")) -> (element=w3888:string[])  [unwired: 1 in]
              n1181 = Insert Into Array(array=w3888, index=0, new element=" " ("new element/subarray")) -> (w3885:string[])
              n1182 = Insert Into Array(array=w3883, index (row)=0, new element=w3885) -> (w3882:string[][])  [unwired: 1 in]
              n1183 = call-poly <vilib>:"Excel Easy Table.vi"("report in"=w3908, "font"=T18 {"font name"="Calibri", "font size"=12.0, "bold"=0, "italic"=0, "underline"=0, "strike through"=0, "font color"=0}, "auto format (none)"=w3917, "start (0, 0)"=cluster{"row":i32, "column":i32} {"row"=0, "column"=0}, "text data"=w3882, "error in (no error)"=w3907) -> ("report out"=w3915:refnum<class "NI_report.lvclass">, "error out"=w3914:errorcluster)  [unwired: 5 in, 3 out]
              n1184 = call-dynamic "Save Report to File.vi"("report in"=w3915, "report file path"=w3919, "error in (no error)"=w3914) -> ()  [unwired: 11 in, 2 out]
            }
          }
          n1185 = local read "Corner Arrays Stbd"() -> (w3377:dbl[][])
          n1186 = local read "Corner Arrays Port"() -> (w3376:dbl[][])
          n1187 = local read "Starboard Arrays"() -> (w3375:dbl[][])
          n1188 = Bundle("x0"=w3464, "dx"=w3463, w3403) -> (w3400:cluster{"x0":dbl, "dx":dbl, dbl[][]})  [unwired: 1 in]
          n1189 = Bundle("x0"=w3468, "dx"=w3467, w3402) -> (w3399:cluster{"x0":dbl, "dx":dbl, dbl[][]})  [unwired: 1 in]
          n1190 = local read "Port Arrays"() -> (w3374:dbl[][])
          n1191 = Bundle("x0"=w3460, "dx"=w3459, w3404) -> (w3458:cluster{"x0":dbl, "dx":dbl, dbl[][]})  [unwired: 1 in]
          n1192 = Array Subset(array=w3471, index (row)=0 ("index"), length (row)=w3373, index (col)=0 ("index"), length (col)=1 ("length")) -> (w3348:string[][])
          n1193 = Array Subset(array=w3471, index (row)=w3373, length (row)=w3372, index (col)=0 ("index"), length (col)=1 ("length")) -> (w3378:string[][])
          n1194 = Array Subset(array=w3471, index (row)=w3371, length (row)=w3370, index (col)=0 ("index"), length (col)=1 ("length")) -> (w3384:string[][])
          n1195 = for {
            tunnel: w3348 -> [w3860] mode=indexing
            tunnel: [w3859] -> w3354 mode=indexing
            n1196 = for {
              tunnel: w3860 -> [w3863] mode=indexing
              tunnel: [w3861] -> w3859 mode=indexing
              n1197 = Concatenate Strings(w3863, "-S" ("string")) -> (w3861:string)
            }
          }
          n1198 = Number To Fractional String(number=w3377, precision (6)=i16 3 ("width (-)")) -> (F-format string=w3396:string[][])  [unwired: 2 in]
          n1199 = Number To Fractional String(number=w3376, precision (6)=i16 3 ("width (-)")) -> (F-format string=w3393:string[][])  [unwired: 2 in]
          n1200 = Build Array (concatenate)(w3404, w3404, w3403, w3402) -> (w3405:dbl[][])
          n1201 = Number To Fractional String(number=w3375, precision (6)=i16 3 ("width (-)")) -> (F-format string=w3390:string[][])  [unwired: 2 in]
          n1202 = Number To Fractional String(number=w3374, precision (6)=i16 3 ("width (-)")) -> (F-format string=w3381:string[][])  [unwired: 2 in]
          n1203 = for {
            tunnel: [w3855] -> w3349 mode=indexing
            tunnel: w3348 -> [w3854] mode=indexing
            n1204 = for {
              tunnel: [w3857] -> w3855 mode=indexing
              tunnel: w3854 -> [w3856] mode=indexing
              n1205 = Concatenate Strings(w3856, "-P" ("string")) -> (w3857:string)
            }
          }
          n1206 = case shown="True" w3450 {
            tunnel: w3666 -> [_ w4029]
            tunnel: w3665 -> [_ w4028]
            tunnel: w3477 -> [_ w4027]
            tunnel: w3399 -> [_ w4026]
            tunnel: w3400 -> [_ w4025]
            tunnel: w3458 -> [_ w4024]
            tunnel: w3457 -> [_ w4023]
            tunnel: w3456 -> [_ w4022]
            frame False {
            }
            frame True {
              # "Sensor Overview"
              "AdB Port" <- w4026
              "AdB Starboard" <- w4025
              "Tach Signal Port" <- w4029
              "Accelerometer Signals Port" <- w4028
              "Tach Signal Stbd" <- w4027
              "Accelerometer Signals Stbd" <- w4023
              "AdB Corners" <- w4024
              "Accelerometer Signals Corners" <- w4022
            }
          }
          n1207 = Array Size(array="MagPhase") -> (size(s)=w3561:i32)
          n1208 = Insert Into Array(array=w3349, index (col)=1 ("disabled index (col)"), new element=w3393) -> (w3346:string[][])  [unwired: 1 in]
          n1209 = Insert Into Array(array=w3354, index (col)=1 ("disabled index (col)"), new element=w3396) -> (w3352:string[][])  [unwired: 1 in]
          n1210 = Insert Into Array(array=w3378, index (col)=1 ("disabled index (col)"), new element=w3390) -> (w3351:string[][])  [unwired: 1 in]
          n1211 = Insert Into Array(array=w3384, index (col)=1 ("disabled index (col)"), new element=w3381) -> (w3345:string[][])  [unwired: 1 in]
          n1212 = for {
            N: w3561 -> [_]
            tunnel: "MagPhase" -> [w4520]
            tunnel: w3405 -> [w4521]
            tunnel: [w4516] -> w3560 mode=indexing
            tunnel: u32[] [4342527, 16728642, 3079936, 46079, 16776704, 14768639, 16753962, 6399, 16728757, 5896447, 0, 16777215, 16711422, 16777215, 16777215, 16777215, 16448250, 16711422, 16777215] -> [w4517] mode=indexing
            i -> [w4519]
            n1213 = flat-sequence {
              tunnel: w4518 -> [w4523]
              tunnel: w4517 -> [w4525]
              frame #0 {
                n1214 = Bundle(w4523, 5) -> (w4522:cluster{i32, i32})  [unwired: 1 in]
                n1215 = property on="MagPhase" class="MCListbox (strict)"("ActiveCell"=w4522) -> ()  [unwired: 2 in, 2 out]
              }
              frame #1 {
                n1216 = property on="MagPhase" class="MCListbox (strict)"("CellBG"=w4525) -> ()  [unwired: 2 in, 2 out]
              }
            }
            n1217 = Index Array(array=w4520, index=w4519) -> (element=w4518:i32)
            n1218 = Index Array(array=w4521, index (row)=w4518) -> (element=w4516:dbl[])  [unwired: 1 in]
          }
          n1219 = Build Array (concatenate)(w3352, w3346, w3351, w3345) -> (w3398:string[][])
          n1220 = Build Array (concatenate)(w3352, w3351) -> (→"Stbd Output Data":string[][])
          n1221 = Build Array (concatenate)(w3346, w3345) -> (→"Port Output Data":string[][])
          n1222 = Index Array(array=w3478, index=0) -> (element=w3565:cluster{"x0":dbl, "dx":dbl, "magnitude":dbl[]})
          n1223 = Unbundle(w3565) -> ("x0"=w3564:dbl, "dx"=w3563:dbl)  [unwired: 1 out]
          n1224 = property on="MagPhase" class="MCListbox (strict)"("ItemNames"=w3398) -> ()  [unwired: 2 in, 2 out]
          n1225 = property on="DAQ Listbox" class="MCListbox (strict)"("ItemNames"=w3398) -> ()  [unwired: 2 in, 2 out]
          n1226 = Bundle("x0"=w3564, "dx"=w3563, w3560) -> (→"Spectrum (AdB)":cluster{"x0":dbl, "dx":dbl, dbl[][]})  [unwired: 1 in]
        }
      }
    }
    n1227 = case "Accelerometer Calibration" shown="True" "Accel Calib Start" {
      tunnel: w366 -> [w3145 _]
      tunnel: "Ship Class" -> [_ w3147]
      frame False {
        n1228 = call-poly <userlib>:"Circular Buffer.vi"("Buffer Size"=w3145, "Operation"=Circular_Buffer_Operations."Initialize") -> ()  [unwired: 6 in, 4 out]
        n1229 = property on="DAQ Start" class="Bool (strict)"("DisabledEnum"=T16."Enabled" ("Disabled")) -> ()  [unwired: 2 in, 2 out]
      }
      frame True {
        # "Enter in the channel list from the excel sheet"
        # "Initialize buffer variable\n1024 samples per channel\n# accelerometer channels"
        # "ignore the first 12 rows because\nthey are the repeated corner accels"
        n1230 = local read "# Accel Channels"() -> (w3148:i32)
        n1231 = local read "# Accel Channels"() -> (w3152:i32)
        n1232 = local read "Sensor Info"() -> (w3161:string[][])
        n1233 = Bundle("Samples per Channel"=u32 1024, "# Accel Channels"=w3148) -> (w3149:T24)  [unwired: 1 in]
        n1234 = while "Write into buffer variable" {
          tunnel: w3149 -> [w3165]
          tunnel: w3147 -> [w3162]
          stop <- w3164 stop-if-true
          n1235 = local read "Accel Calib Start"() -> (w3163:bool)
          n1236 = Not(x=w3163) -> (.not. x?=w3164:bool)
          n1237 = case shown="\"LA Class\"" w3162 {
            tunnel: [w3169 w3170 w3173] -> w3166
            tunnel: w3164 -> [w3168 w3171 w3172]
            frame "Simulated Signals Ohio", Default {
              n1238 = call "DAQ Assistant Accel Calib Ohio2"("stop (F)"=w3168) -> ("data"=w3169:dynamicdata)  [unwired: 15 in, 3 out]
            }
            frame "LA Class" {
              n1239 = call "DAQ Assistant Accel Calib LAclass"("stop (F)"=w3171) -> ("data"=w3170:dynamicdata)  [unwired: 15 in, 3 out]
            }
            frame "Ohio Class" {
              n1240 = call "DAQ Assistant Accel Calib Ohio"("stop (F)"=w3172) -> ("data"=w3173:dynamicdata)  [unwired: 15 in, 3 out]
            }
          }
          n1241 = call-poly <userlib>:"Circular Buffer.vi"("Buffer Size"=w3165, "Operation"=Circular_Buffer_Operations."Write", "Data In"=w3166) -> ()  [unwired: 5 in, 4 out]
        }
        n1242 = call-poly <userlib>:"Circular Buffer.vi"("Buffer Size"=w3149, "Operation"=Circular_Buffer_Operations."Initialize") -> ()  [unwired: 6 in, 4 out]
        n1243 = Array Subset(array=w3161, index (row)=0 ("index"), length (row)=w3152, index (col)=0 ("index"), length (col)=2 ("length")) -> (w3151:string[][])
        n1244 = Insert Into Array(array=w3151, index (col)=2 ("disabled index (col)"), new element=string[] ["", "", "", "", "", "", "", "", "", "", "", "", "", "", "", "", "", "", "", "", "", "", "", "", "", "", "", "", "", "", " ", "", "", "", "", "", "", "", "", "", ""] ("new element/subarray")) -> (w3160:string[][])  [unwired: 1 in]
        n1245 = property on="DAQ Start" class="Bool (strict)"("DisabledEnum"=T16."Disabled and Grayed Out" ("Disabled")) -> ()  [unwired: 2 in, 2 out]
        n1246 = property on="Calibration Channel List" class="MCListbox (strict)"("ItemNames"=w3160) -> ()  [unwired: 2 in, 2 out]
        n1247 = while "Read from buffer, Write calibration values" {
          tunnel: w3149 -> [w3177]
          stop <- w3184 stop-if-true
          n1248 = Unbundle(w3177) -> ("Samples per Channel"=w3176:u32)  [unwired: 1 out]
          n1249 = local read "Accel Calib Start"() -> (w3175:bool)
          n1250 = Not(x=w3175) -> (.not. x?=w3184:bool)
          n1251 = call-poly <userlib>:"Circular Buffer.vi"("Buffer Size"=w3177, "Read Size"=w3176, "Operation"=Circular_Buffer_Operations."Read (most recent)") -> ("Data Out"=w3174:waveform(dbl)[])  [unwired: 5 in, 3 out]
          n1252 = call "Convert from Dynamic Data3"("Dynamic Data Type"=w3174) -> ("Array"=w3179:dbl[][])  [unwired: 3 in]
          n1253 = Array Size(array=w3179) -> (size(s)=w3182:i32[])
          n1254 = Equal?(x=w3182, y=w3176) -> (x = y?=w3180:bool[])
          n1255 = Index Array(array=w3180, index=1) -> (element=w3178:bool)
          n1256 = case shown="True" w3178 {
            tunnel: w3174 -> [_ w3187]
            frame False {
            }
            frame True {
              # "Should read 4V\npeak when calibrator\nis running"
              n1257 = Replace Array Subset(array=bool[] [FALSE, FALSE, FALSE, FALSE, FALSE, FALSE, FALSE, FALSE, FALSE, FALSE, FALSE, FALSE, FALSE, FALSE, FALSE, FALSE, FALSE, FALSE, FALSE, FALSE, FALSE, FALSE, FALSE, FALSE, FALSE, FALSE, FALSE, FALSE, FALSE, FALSE, FALSE, FALSE, FALSE, FALSE, FALSE, FALSE, FALSE, FALSE, FALSE, FALSE], new element=TRUE ("new element/subarray"), index="Calibration Channel List") -> (w3201:bool[])
              n1258 = call "Convert to Dynamic Data25"("Array"=w3201) -> ("Dynamic Data Type"=w3200:dynamicdata)  [unwired: 3 in]
              n1259 = call "Select Signals2"("Selector Input"=w3200, "Signals"=w3187) -> ("Signal Out"=w3198:dynamicdata)  [unwired: 8 in, 1 out]
              n1260 = case shown="True" "Calib Avg" {
                tunnel: [u32 10 ("number of averages") u32 1000 ("number of averages")] -> w3186
                frame False {
                }
                frame True {
                }
              }
              n1261 = Divide(x=w3198, y=0.004) -> (x/y=w3192:dynamicdata)
              n1262 = call "Power Spectrum16"("input signals"=w3192, "number of averages"=w3186) -> ("spectra"=w3191:cluster{"x0":dbl, "dx":dbl, "magnitude":dbl[]}[])  [unwired: 12 in, 5 out]
              "FFT mV/in/s" <- w3191
              n1263 = Multiply(x=w3198, y=10.0) -> (x*y=w3197:dynamicdata)
              "Volts Graph" <- w3197
              n1264 = Index Array(array=w3191, index=0) -> (element=w3189:cluster{"x0":dbl, "dx":dbl, "magnitude":dbl[]})
